vi "Not Equal.vi"   [LabVIEW 2017, in "NI_Matrix.lvlib"]
doc: "Returns TRUE if <B>x</B> is not equal to <B>y</B>. Otherwise, this function returns FALSE."
uses:
  <vilib>/Analysis/Matrix/NI_Matrix.lvlib
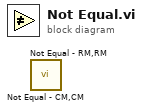
[diagram p0: block diagram]
diagram:
  n1 = call <vilib>:"Not Equal - CM,CM.vi"() -> ()  [unwired: 2 in, 1 out]
  n2 = call <vilib>:"Not Equal - RM,RM.vi"() -> ()  [unwired: 2 in, 1 out]
